vi "3D Robot Simulator.vi"() -> ()   [LabVIEW 2021]
uses:
  <vilib>/Utility/miscctls.llb/LV3DPointTypeDef.ctl
  <vilib>/picture/3D Picture Control/Object/Create Object (drawable).vi
  <vilib>/picture/3D Picture Control/Object/Add Object (no reference).vi
  <vilib>/picture/3D Picture Control/NI_3D Picture Control.lvlib
panel:
  out "Waveform Graph":u32[](graph)
  out "Query Time (ms)":u32
  in  "Log Mode":bool=TRUE
  out "FROM NN MODEL\nRobot OK":bool
  out "Elapesed Time(s)":dbl
  in  "Delay (ms)":u32=50
  in  "Sim Mode":bool
  out "Ball 2 Position":T1
  out "Ball 1 Position":T1
  out "Arm Base Position":T1
  in  "Z axis deg":sgl(slide) min=0 max=360 step=1 scale=0.0..360.0
  in  "Y axis deg":sgl(slide) min=0 max=360 step=1 scale=0.0..360.0
  in  "Euler Rotation":sgl(slide) min=0 max=360 step=1 scale=0.0..360.0
  in  "X axis deg":sgl(slide) min=0 max=360 step=1 scale=0.0..360.0
  in  "Wall":dbl(slide)=0.5 min=0.0 max=1.0 step=0.05 scale=0.0..1.0
  in  "Background":u32(colorbox)=4868682
  in  "Axis Color":u32(colorbox)=16777225
  in  "Wall Color":u32(colorbox)=6618880
  in  "Machine Color":u32(colorbox)=16777226
  out "Test Area":refnum<vi>(3d-picture)
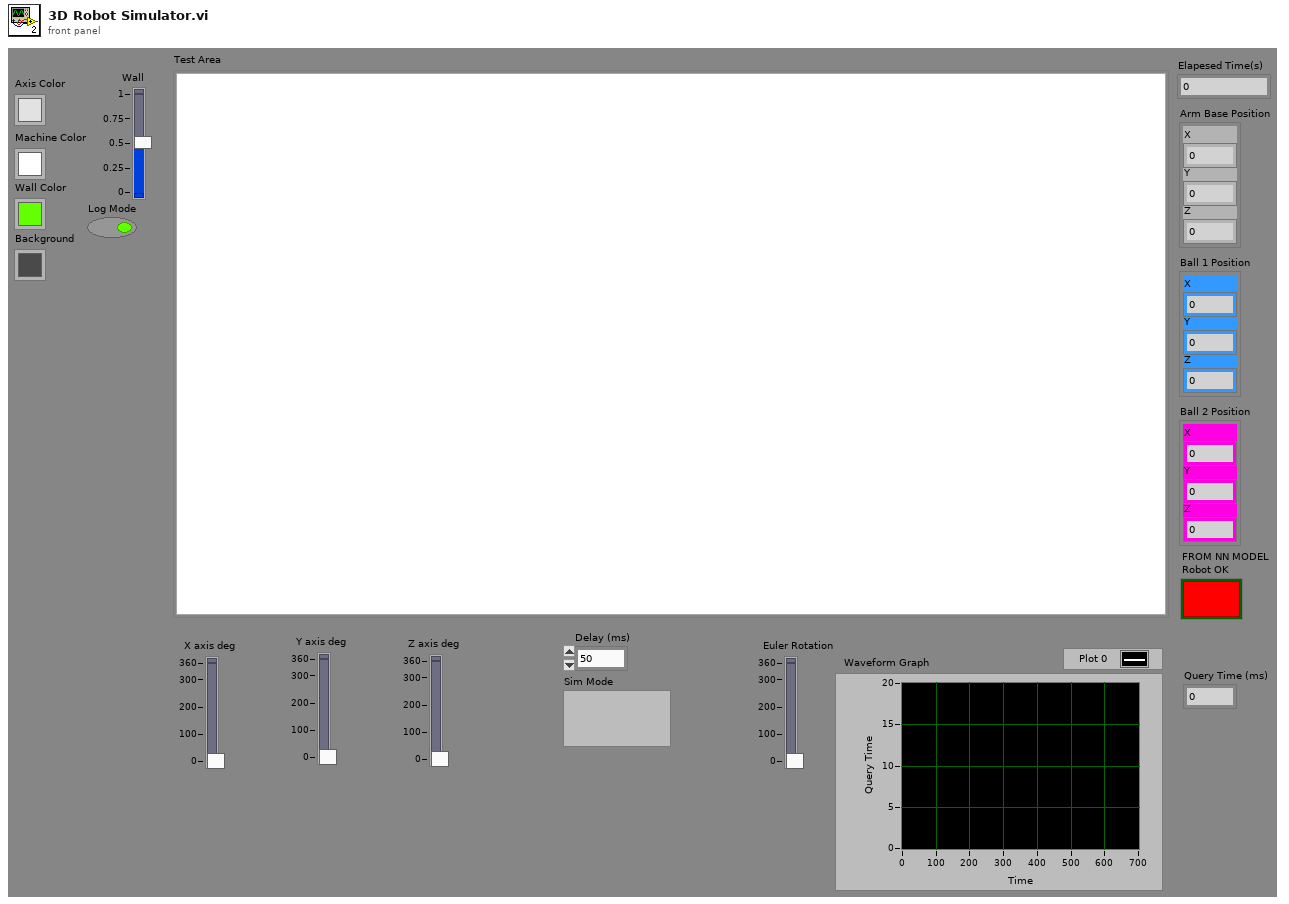
[diagram p1: front panel]
types:
  T1 = typedef "LV3DPointTypeDef.ctl" = cluster{"X":sgl, "Y":sgl, "Z":sgl}
  T2 = cluster{"Ball1OK":bool, "Ball2OK":bool, "BothOK":dbl, "StartTime":u32}
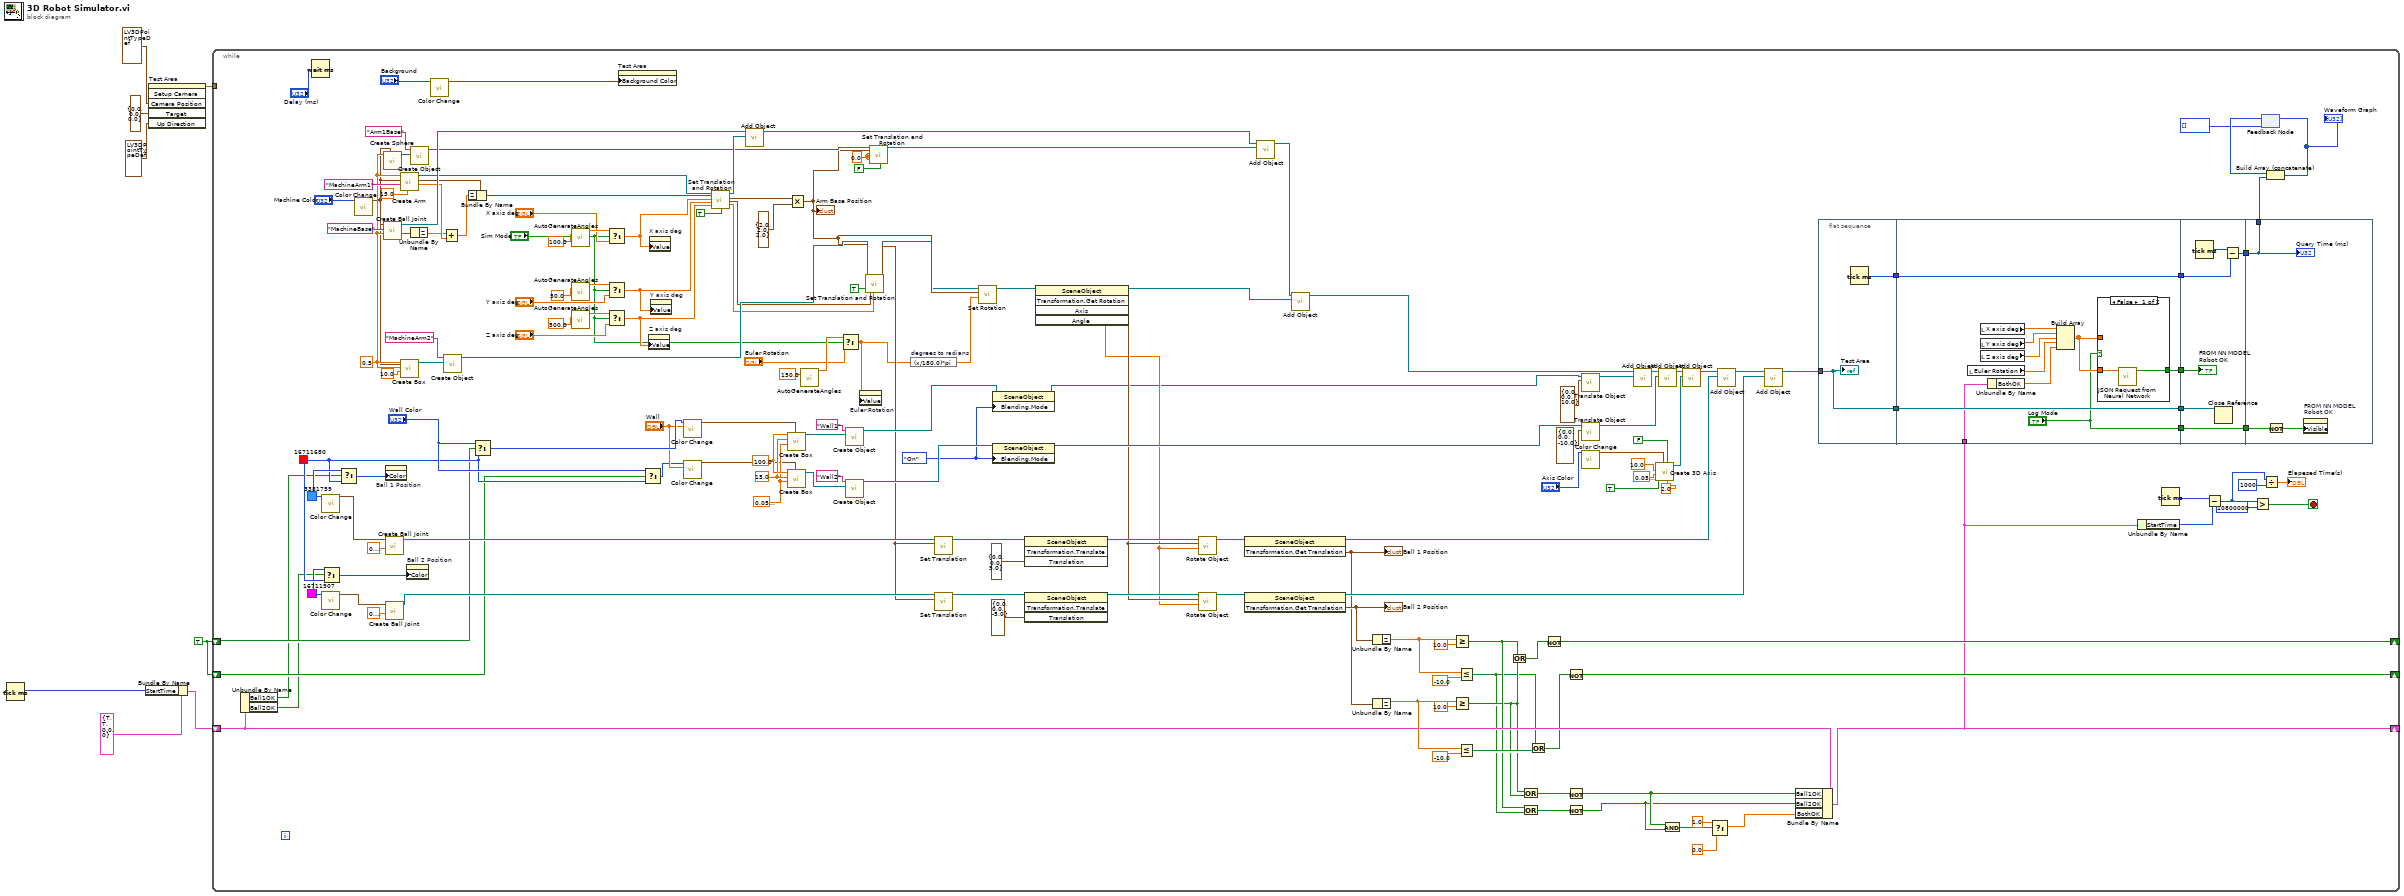
[diagram p0: block diagram]
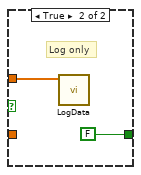
[diagram p2: hidden frame]
diagram:
  w4 = TRUE
  n1 = Tick Count (ms)() -> (millisecond timer value=w3:u32)
  n2 = Bundle By Name(cluster=T2 {"Ball1OK"=TRUE, "Ball2OK"=TRUE, "BothOK"=0.0, "StartTime"=0}, "StartTime"=w3) -> (w1:T2)
  n3 = invoke on="Test Area" class="SceneGraphDisp (strict)" method="Setup Camera"("Camera Position"=T1 {"X"=25.4, "Y"=40.2, "Z"=20.3}, "Target"=T1 {"X"=0.0, "Y"=0.0, "Z"=0.0}, "Up Direction"=T1 {"X"=0.2, "Y"=0.3, "Z"=0.4}) -> (error out=w5:errorcluster)  [unwired: 3 in, 5 out]
  n4 = while {
    tunnel: w5 -> [_]
    shift-right: [w84] -> _
    shift-left: w4 -> [w44]
    shift-right: [w75] -> _
    shift-left: w4 -> [w45]
    shift-right: [w26] -> _
    shift-left: w1 -> [w41]
    stop <- w22 stop-if-true
    w46 = u32 16711907 ("Color")
    w47 = u32 16711680 ("Wall Color")
    w88 = sgl 0.0 ("X axis deg")
    w48 = u32 3381759 ("Color")
    w116 = sgl 0.5 ("Radius 2")
    w148 = enum16{"Inherit Value", "Off", "On"}."On" ("Blending:Mode")
    w162 = sgl 0.05 ("Length X")
    w163 = sgl 15.0 ("Length X")
    w164 = sgl 100.0 ("Length X")
    n5 = Unbundle By Name(w41) -> ("Ball1OK"=w43:bool, "Ball2OK"=w42:bool)
    n6 = Wait (ms)(milliseconds to wait="Delay (ms)") -> ()  [unwired: 1 out]
    n7 = call <vilib>:"Color Change.vi"("Color"=w48) -> ("RGBA"=w104:cluster{"R":sgl, "G":sgl, "B":sgl, "A":sgl})  [unwired: 10 in]
    n8 = call <vilib>:"Color Change.vi"("Color"=w46) -> ("RGBA"=w51:cluster{"R":sgl, "G":sgl, "B":sgl, "A":sgl})  [unwired: 10 in]
    n9 = Select(t=w46, s=w42, f=w47) -> (s? t:f=w49:u32)
    n10 = Select(t=w48, s=w43, f=w47) -> (s? t:f=w50:u32)
    n11 = call <vilib>:"Color Change.vi"("Color"="Machine Color") -> ("RGBA"=w113:cluster{"R":sgl, "G":sgl, "B":sgl, "A":sgl})  [unwired: 10 in]
    n12 = call <vilib>:"Create Sphere.vi"("Color"=w113, "Radius"=w116) -> ("New Sphere Refnum"=w139:refnum<vi>)  [unwired: 8 in, 1 out]
    n13 = call "Create Ball Joint.vi"("Radius 2"=w116, "Name"="MachineBase", "RGBA"=w113) -> ("Transformation.GetTranslation"=w127:T1, "SceneObject out"=w146:refnum<vi>)  [unwired: 7 in]
    n14 = property on="Ball 1 Position" class="Clust (strict)"("Color"=w50) -> ()  [unwired: 2 in, 2 out]
    n15 = call "Create Ball Joint.vi"("Radius 2"=sgl 0.6, "RGBA"=w104) -> ("SceneObject out"=w115:refnum<vi>)  [unwired: 8 in, 1 out]
    n16 = call "Create Ball Joint.vi"("Radius 2"=sgl 0.6, "RGBA"=w51) -> ("SceneObject out"=w103:refnum<vi>)  [unwired: 8 in, 1 out]
    n17 = call "Create Arm.vi"("Length"=sgl 15.0 ("Length Z"), "Name"="MachineArm1", "Color"=w113, "Radius"=w116) -> ("Half Length"=w140:sgl, "Transformation.GetTranslation"=w144:T1, "SceneObject out"=w145:refnum<vi>)  [unwired: 5 in]
    n18 = call <vilib>:"Create Box.vi"("Color"=w113, "Length Z"=sgl 10.0, "Length Y"=w116, "Length X"=w116) -> ("New Box Refnum"=w132:refnum<vi>)  [unwired: 6 in, 1 out]
    n19 = property on="Ball 2 Position" class="Clust (strict)"("Color"=w49) -> ()  [unwired: 2 in, 2 out]
    n20 = call-poly <vilib>:"Create Object.vi"("Geometry"=w139, "Name"="Arm1Base") -> ("Scene:New Object"=w130:refnum<vi>)  [unwired: 8 in, 1 out]
    n21 = Unbundle By Name(w127) -> ("Z"=w126:sgl)
    n22 = call <vilib>:"Color Change.vi"("Color"="Background") -> ("RGBA"=w154:cluster{"R":sgl, "G":sgl, "B":sgl, "A":sgl})  [unwired: 10 in]
    n23 = Add(x=w126, y=w140) -> (x+y=w142:sgl)
    n24 = call-poly <vilib>:"Create Object.vi"("Geometry"=w132, "Name"="MachineArm2") -> ("Scene:New Object"=w123:refnum<vi>)  [unwired: 8 in, 1 out]
    n25 = Bundle By Name(cluster=w144, "Z"=w142) -> (w143:T1)
    n26 = Select(t="Wall Color", s=w44, f=w47) -> (s? t:f=w83:u32)
    n27 = call "AutoGenerateAngles.vi"("Randomization Reset"=100.0) -> ("Value"=w68:dbl)  [unwired: 14 in]
    n28 = call "AutoGenerateAngles.vi"("Randomization Reset"=50.0) -> ("Value"=w64:dbl)  [unwired: 14 in]
    n29 = call "AutoGenerateAngles.vi"("Randomization Reset"=500.0) -> ("Value"=w62:dbl)  [unwired: 14 in]
    n30 = Select(t=w68, s="Sim Mode", f="X axis deg") -> (s? t:f=w59:dbl)
    n31 = Select(t=w64, s="Sim Mode", f="Y axis deg") -> (s? t:f=w58:dbl)
    n32 = Select(t=w62, s="Sim Mode", f="Z axis deg") -> (s? t:f=w57:dbl)
    n33 = property on="Test Area" class="SceneGraphDisp (strict)"("Background Color"=w154) -> ()  [unwired: 2 in, 2 out]
    n34 = Select(t="Wall Color", s=w45, f=w47) -> (s? t:f=w76:u32)
    n35 = property on="Z axis deg" class="Slide (strict)"("Value"=w57) -> ()  [unwired: 2 in, 2 out]
    n36 = property on="X axis deg" class="Slide (strict)"("Value"=w59) -> ()  [unwired: 2 in, 2 out]
    n37 = property on="Y axis deg" class="Slide (strict)"("Value"=w58) -> ()  [unwired: 2 in, 2 out]
    n38 = call <vilib>:"Color Change.vi"("Alpha"="Wall", "Color"=w83) -> ("RGBA"=w158:cluster{"R":sgl, "G":sgl, "B":sgl, "A":sgl})  [unwired: 9 in]
    n39 = call <vilib>:"Color Change.vi"("Alpha"="Wall", "Color"=w76) -> ("RGBA"=w79:cluster{"R":sgl, "G":sgl, "B":sgl, "A":sgl})  [unwired: 9 in]
    n40 = call "Set Translation and Rotation.vi"("SceneObject in"=w145, "Transformation.GetTranslation in"=w143, "X axis deg"=w59, "Y axis deg"=w58, "Z axis deg"=w57, "Relative?"=TRUE) -> ("SceneObject out"=w137:refnum<vi>, "Transformation.GetTranslation out"=w120:T1, "Rotation Axis Out"=w119:T1, "Angle Out"=w117:sgl)  [unwired: 10 in]
    n41 = call-poly <vilib>:"Add Object.vi"("New Object In"=w137, "Scene Object In"=w146) -> ("Scene Object Out"=w136:refnum<vi>)  [unwired: 8 in, 1 out]
    n42 = call <vilib>:"Create Box.vi"("Color"=w158, "Length Z"=w162, "Length Y"=w163, "Length X"=w164) -> ("New Box Refnum"=w165:refnum<vi>)  [unwired: 6 in, 1 out]
    n43 = call <vilib>:"Create Box.vi"("Color"=w79, "Length Z"=w162, "Length Y"=w163, "Length X"=w164) -> ("New Box Refnum"=w151:refnum<vi>)  [unwired: 6 in, 1 out]
    n44 = Multiply(x=w120, y=T1 {"X"=2.0, "Y"=2.0, "Z"=2.0}) -> (x*y=w122:T1)
    "Arm Base Position" <- w122
    n45 = call "AutoGenerateAngles.vi"("Randomization Reset"=150.0) -> ("Value"=w55:dbl)  [unwired: 14 in]
    n46 = Select(t=w55, s="Sim Mode", f="Euler Rotation") -> (s? t:f=w52:dbl)
    n47 = call-poly <vilib>:"Create Object.vi"("Geometry"=w165, "Name"="Wall1") -> ("Scene:New Object"=w152:refnum<vi>)  [unwired: 8 in, 1 out]
    n48 = call-poly <vilib>:"Create Object.vi"("Geometry"=w151, "Name"="Wall2") -> ("Scene:New Object"=w150:refnum<vi>)  [unwired: 8 in, 1 out]
    n49 = property on="Euler Rotation" class="Slide (strict)"("Value"=w52) -> ()  [unwired: 2 in, 2 out]
    n50 = call "Set Translation and Rotation.vi"("SceneObject in"=w123, "Transformation.GetTranslation in"=w122, "Initial Rotation Axis"=w119, "Initial Rotation Angle"=w117, "Relative?"=TRUE) -> ("SceneObject out"=w91:refnum<vi>, "Transformation.GetTranslation out"=w98:T1)  [unwired: 11 in, 2 out]
    n51 = call "Set Translation and Rotation.vi"("SceneObject in"=w130, "Transformation.GetTranslation in"=w122, "X axis deg"=w88, "Y axis deg"=w88, "Z axis deg"=w88, "Relative?"=FALSE) -> ("SceneObject out"=w135:refnum<vi>)  [unwired: 10 in, 3 out]
    n52 = expression code="(x/180.0)*pi" "degrees to radians"(w52) -> (w90:dbl)
    n53 = call <vilib>:"Set Translation.vi"("Translation"=w98, "Scene Object"=w115) -> ("Translated Object"=w111:refnum<vi>)  [unwired: 8 in, 1 out]
    n54 = call <vilib>:"Set Translation.vi"("Translation"=w98, "Scene Object"=w103) -> ("Translated Object"=w106:refnum<vi>)  [unwired: 8 in, 1 out]
    n55 = call <vilib>:"Set Rotation.vi"("Angle"=w90, "Axis"=w122, "Scene Object"=w91) -> ("Rotated Scene Object"=w89:refnum<vi>)  [unwired: 7 in, 1 out]
    n56 = property class="SceneObject"(reference=w152, "Blending.Mode"=w148) -> (reference out=w85:refnum<vi>)  [unwired: 1 in, 1 out]
    n57 = property class="SceneObject"(reference=w150, "Blending.Mode"=w148) -> (reference out=w149:refnum<vi>)  [unwired: 1 in, 1 out]
    n58 = invoke class="SceneObject" method="Transformation.Translate"(reference=w111, "Translation"=T1 {"X"=0.0, "Y"=0.0, "Z"=5.0} ("y")) -> (reference out=w109:refnum<vi>)  [unwired: 2 in, 3 out]
    n59 = invoke class="SceneObject" method="Transformation.Translate"(reference=w106, "Translation"=T1 {"X"=0.0, "Y"=0.0, "Z"=-5.0} ("y")) -> (reference out=w108:refnum<vi>)  [unwired: 2 in, 3 out]
    n60 = invoke class="SceneObject" method="Transformation.Get Rotation"(reference=w89) -> (reference out=w121:refnum<vi>, "Axis"=w102:T1, "Angle"=w101:sgl)  [unwired: 4 in, 2 out]
    n61 = call <vilib>:"Rotate Object.vi"("Angle"=w101, "Axis"=w102, "Scene.Object In"=w109) -> ("Scene.Object Out"=w96:refnum<vi>)  [unwired: 7 in, 1 out]
    n62 = call <vilib>:"Rotate Object.vi"("Angle"=w101, "Axis"=w102, "Scene.Object In"=w108) -> ("Scene.Object Out"=w94:refnum<vi>)  [unwired: 7 in, 1 out]
    n63 = invoke class="SceneObject" method="Transformation.Get Translation"(reference=w96) -> (reference out=w95:refnum<vi>, "Transformation.GetTranslation"=w74:T1)  [unwired: 2 in, 1 out]
    "Ball 1 Position" <- w74
    n64 = invoke class="SceneObject" method="Transformation.Get Translation"(reference=w94) -> (reference out=w93:refnum<vi>, "Transformation.GetTranslation"=w82:T1)  [unwired: 2 in, 1 out]
    "Ball 2 Position" <- w82
    n65 = call-poly <vilib>:"Add Object.vi"("New Object In"=w135, "Scene Object In"=w136) -> ("Scene Object Out"=w129:refnum<vi>)  [unwired: 8 in, 1 out]
    n66 = call-poly <vilib>:"Add Object.vi"("New Object In"=w121, "Scene Object In"=w129) -> ("Scene Object Out"=w128:refnum<vi>)  [unwired: 8 in, 1 out]
    n67 = Unbundle By Name(w82) -> ("Z"=w81:sgl)
    n68 = Unbundle By Name(w74) -> ("Z"=w71:sgl)
    n69 = Greater Or Equal?(x=w81, y=10.0) -> (x >= y?=w37:bool)
    n70 = Greater Or Equal?(x=w71, y=10.0) -> (x >= y?=w36:bool)
    n71 = Less Or Equal?(x=w81, y=-10.0) -> (x <= y?=w35:bool)
    n72 = Less Or Equal?(x=w71, y=-10.0) -> (x <= y?=w69:bool)
    n73 = Or(x=w37, y=w36) -> (x .or. y?=w70:bool)
    n74 = Or(x=w36, y=w36) -> (x .or. y?=w38:bool)
    n75 = Or(x=w37, y=w35) -> (x .or. y?=w39:bool)
    n76 = Or(x=w35, y=w69) -> (x .or. y?=w40:bool)
    n77 = Not(x=w70) -> (.not. x?=w84:bool)
    n78 = Not(x=w40) -> (.not. x?=w75:bool)
    n79 = Not(x=w38) -> (.not. x?=w32:bool)
    n80 = Not(x=w39) -> (.not. x?=w31:bool)
    n81 = call <vilib>:"Translate Object.vi"("Translation"=cluster{"X":sgl, "Y":sgl, "Z":sgl} {"X"=0.0, "Y"=0.0, "Z"=10.0}, "Scene.Object In"=w85) -> ("Scene.Object Out"=w175:refnum<vi>)  [unwired: 8 in, 1 out]
    n82 = call <vilib>:"Translate Object.vi"("Translation"=cluster{"X":sgl, "Y":sgl, "Z":sgl} {"X"=0.0, "Y"=0.0, "Z"=-10.0}, "Scene.Object In"=w149) -> ("Scene.Object Out"=w173:refnum<vi>)  [unwired: 8 in, 1 out]
    n83 = call <vilib>:"Color Change.vi"("Color"="Axis Color") -> ("RGBA"=w156:cluster{"R":sgl, "G":sgl, "B":sgl, "A":sgl})  [unwired: 10 in]
    n84 = call-poly <vilib>:"Add Object.vi"("New Object In"=w175, "Scene Object In"=w128) -> ("Scene Object Out"=w174:refnum<vi>)  [unwired: 8 in, 1 out]
    n85 = call <vilib>:"Create 3D Axis.vi"("Character Size"=sgl 2.0, "Half plane?"=FALSE, "Axis label?"=TRUE, "Color"=w156, "Radius"=sgl 0.05, "Length"=sgl 10.0) -> ("New Object Refnum"=w170:refnum<vi>)  [unwired: 4 in, 1 out]
    n86 = call-poly <vilib>:"Add Object.vi"("New Object In"=w173, "Scene Object In"=w174) -> ("Scene Object Out"=w124:refnum<vi>)  [unwired: 8 in, 1 out]
    n87 = And(x=w32, y=w31) -> (x .and. y?=w30:bool)
    n88 = call-poly <vilib>:"Add Object.vi"("New Object In"=w170, "Scene Object In"=w124) -> ("Scene Object Out"=w114:refnum<vi>)  [unwired: 8 in, 1 out]
    n89 = Select(t=1.0, s=w30, f=0.0 ("t")) -> (s? t:f=w27:dbl)
    n90 = call-poly <vilib>:"Add Object.vi"("New Object In"=w95, "Scene Object In"=w114) -> ("Scene Object Out"=w100:refnum<vi>)  [unwired: 8 in, 1 out]
    n91 = call-poly <vilib>:"Add Object.vi"("New Object In"=w93, "Scene Object In"=w100) -> ("Scene Object Out"=w99:refnum<vi>)  [unwired: 8 in, 1 out]
    n92 = Bundle By Name(cluster=w41, "Ball1OK"=w32, "Ball2OK"=w31, "BothOK"=w27) -> (w26:T2)
    n93 = flat-sequence {
      tunnel: w99 -> [w177]
      tunnel: [w177] -> w34
      tunnel: [w176] -> w14
      tunnel: w34 -> [w188]
      tunnel: [w188] -> w33
      tunnel: w26 -> [w187]
      tunnel: [w181] -> w18
      tunnel: ["Log Mode"] -> w16
      tunnel: [w178] -> w15
      tunnel: w14 -> [w178]
      tunnel: w33 -> [w198]
      tunnel: w18 -> [w197]
      tunnel: [w196] -> w17
      tunnel: w16 -> [w196]
      tunnel: w15 -> [w194]
      tunnel: [w193] -> w13
      tunnel: w17 -> [w201]
      tunnel: w13 -> [w199]
      tunnel: [w199] -> w12
      frame #0 {
        n94 = Tick Count (ms)() -> (millisecond timer value=w176:u32)
        "Test Area" <- w177
      }
      frame #1 {
        n95 = local read "Euler Rotation"() -> (w183:sgl)
        n96 = local read "X axis deg"() -> (w186:sgl)
        n97 = local read "Y axis deg"() -> (w185:sgl)
        n98 = local read "Z axis deg"() -> (w184:sgl)
        n99 = Unbundle By Name(w187) -> ("BothOK"=w182:dbl)
        n100 = Build Array(w186, w185, w184, w183, w182) -> (w180:dbl[])
        n101 = case shown="False" "Log Mode" {
          tunnel: w180 -> [w190 _]
          tunnel: [w189 FALSE ("x != 0?")] -> w181
          tunnel: w180 -> [_ w191]
          frame False {
            n102 = call "JSON Request from Neural Network.vi"("Features"=w190) -> ("x != 0?"=w189:bool)  [unwired: 9 in, 1 out]
          }
          frame True {
            # "Log only"
            n103 = call "LogData.vi"("1D data"=w191) -> ()  [unwired: 11 in]
          }
        }
      }
      frame #2 {
        n104 = Tick Count (ms)() -> (millisecond timer value=w195:u32)
        n105 = Close Reference(reference=w198) -> ()  [unwired: 1 in, 1 out]
        n106 = Subtract(x=w195, y=w194) -> (x-y=w193:u32)
        "FROM NN MODEL\nRobot OK" <- w197
      }
      frame #3 {
        n107 = Not(x=w201) -> (.not. x?=w200:bool)
        n108 = property on="FROM NN MODEL\nRobot OK" class="Bool (strict)"("Visible"=w200) -> ()  [unwired: 2 in, 2 out]
        "Query Time (ms)" <- w199
      }
    }
    n109 = Unbundle By Name(w26) -> ("StartTime"=w24:u32)
    n110 = Tick Count (ms)() -> (millisecond timer value=w25:u32)
    n111 = Subtract(x=w25, y=w24) -> (x-y=w21:u32)
    n112 = Greater?(x=w21, y=u32 10800000) -> (0:w22:bool)
    n113 = feedback #1(u32[] []) -> (w11:u32[])
    n114 = Divide(x=w21, y=u32 1000) -> (x/y=→"Elapesed Time(s)":dbl)
    n115 = Build Array (concatenate)(w11, w12) -> (w9:u32[])
    "Waveform Graph" <- w9
    n116 = feedback-in #1(w9) -> ()
  }
